vi "ImageInit.vi"(11 "path":string) -> (0 "error out":errorcluster, 4 "return":i32)   [LabVIEW 2015]
uses:
  [Global] Image.vi
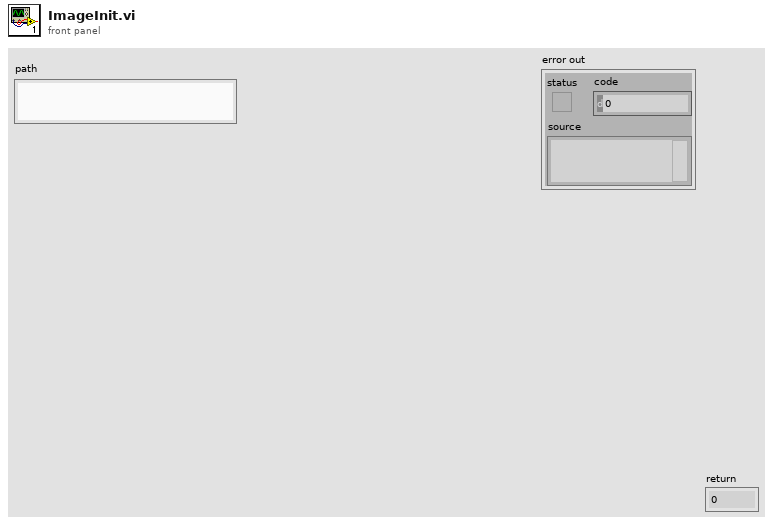
[diagram p1: front panel]
types:
  T1 = typedef "Image Type" = u32
  T2 = typedef "IMAQ Image.ctl" = refnum<image>
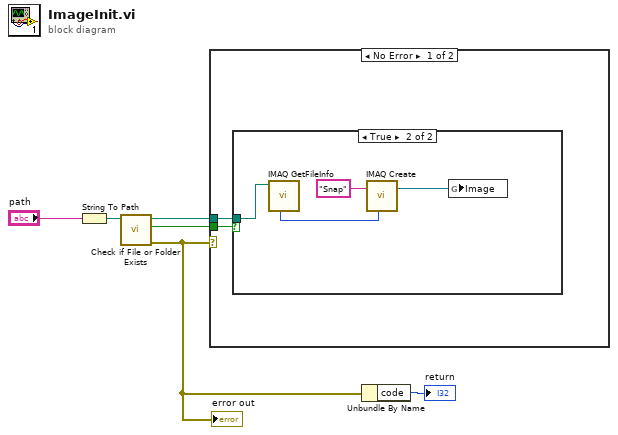
[diagram p0: block diagram]
diagram:
  n1 = String To Path(string="path") -> (path=w5:path)
  n2 = call <vilib>:"Check if File or Folder Exists.vi"("path"=w5) -> ("error out"=w1:errorcluster, "file or folder exists?"=w4:bool, "dup path"=w3:path)  [unwired: 8 in]
  "error out" <- w1
  n3 = case shown="No Error" w1 {
    tunnel: w4 -> [w8 _]
    tunnel: w3 -> [w7 _]
    frame No Error {
      n4 = case shown="True" w8 {
        tunnel: w7 -> [_ w10]
        frame False {
        }
        frame True {
          n5 = call "IMAQ GetFileInfo"("File Path"=w10) -> ("Image Type"=w11:T1)  [unwired: 4 in, 6 out]
          n6 = call "IMAQ Create"("Image Name"="Snap", "Image Type"=w11) -> ("New Image"=w9:T2)  [unwired: 2 in, 2 out]
          n7 = global write "[Global] Image.vi" "Image"(w9) -> ()
        }
      }
    }
    frame Error {
    }
  }
  n8 = Unbundle By Name(w1) -> ("code"=→"return":i32)
